vi "nicrioDebugToken.vi"() -> ()   [LabVIEW 2017]
panel:
  out "text":string
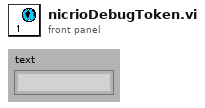
[diagram p1: front panel]
diagram:
